vi "SelectMessages.vi"(8 "error in (no error)":errorcluster, 11 "Messages in":T1[](array[typedef])) -> (0 "error out":errorcluster, 2 "Cancelled":bool, 3 "Messages out":T1[](array[typedef]))   [LabVIEW 2017, in "MessageGen.lvlib"]
uses:
  <vilib>/addons/InsightCM/MessageBus/CodeGen/MessageGen.lvlib
  <vilib>/addons/InsightCM/MessageBus/CodeGen/controls/MessageData.ctl
  <vilib>/addons/InsightCM/MessageBus/CodeGen/controls/MessageType.ctl
  <vilib>/addons/InsightCM/MessageBus/CodeGen/controls/Parameter.ctl
  <vilib>/addons/InsightCM/MessageBus/CodeGen/controls/ParameterType.ctl
panel:
  in  "DelectAll":bool
  in  "SelectAll":bool
  in  "Cancel":bool
  in  "Ok":bool
  in  "Messages":cluster{"Boolean":bool, "String":string}[](array[cluster])
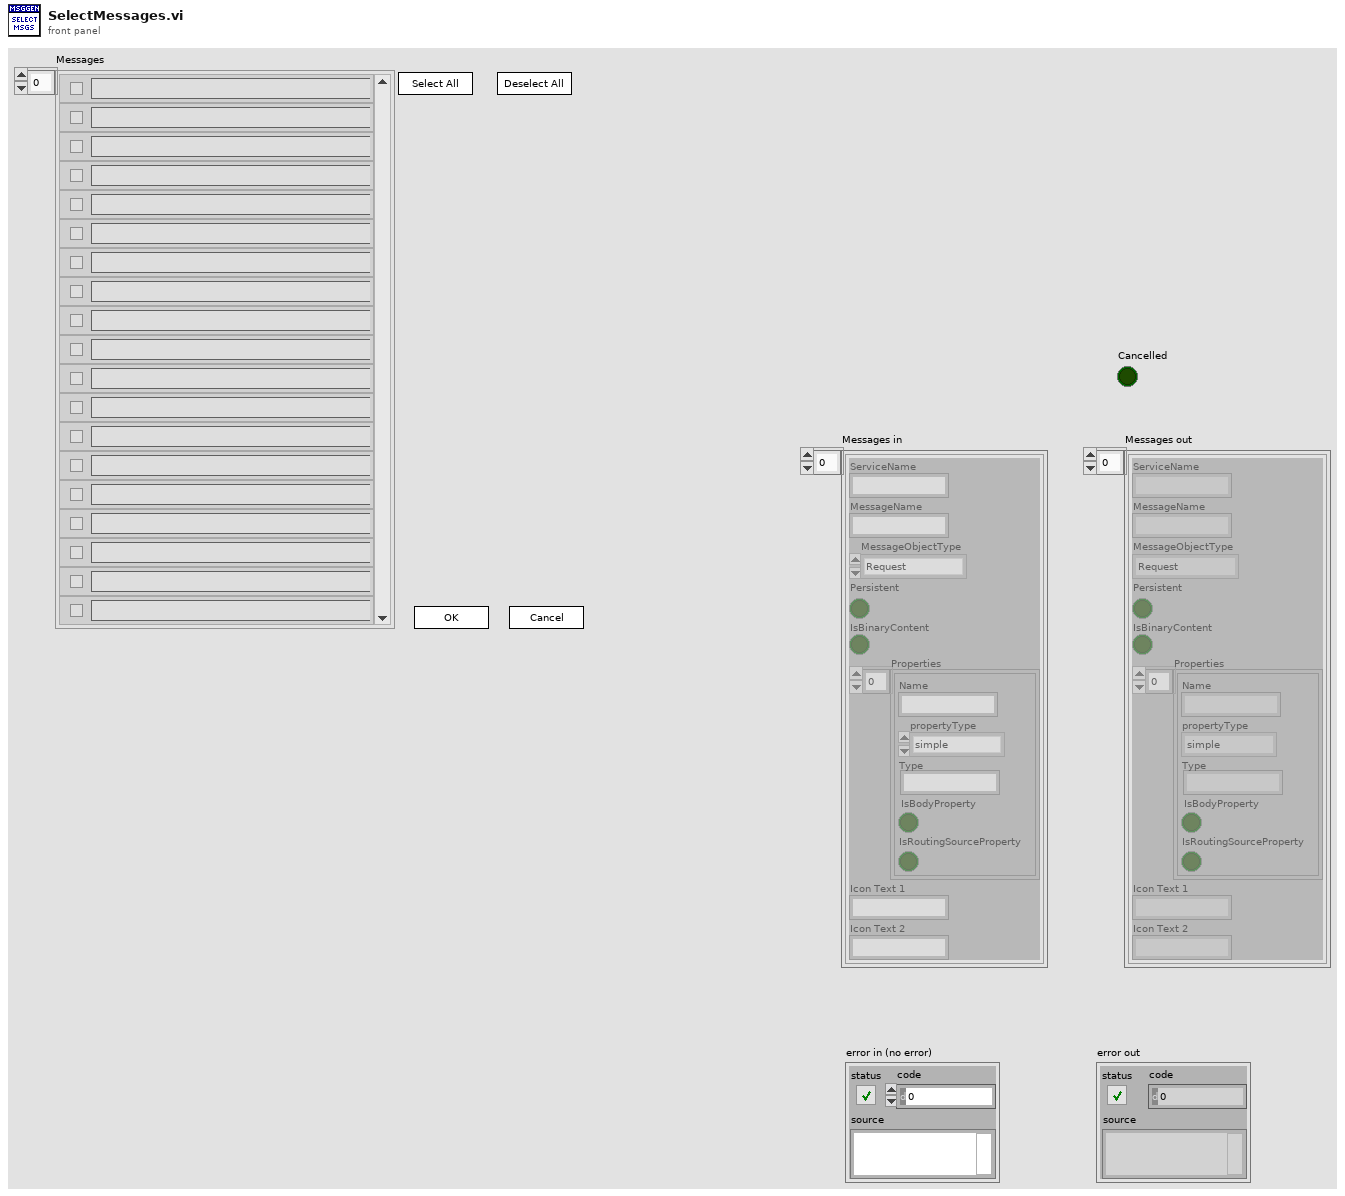
[diagram p1: front panel]
types:
  T1 = typedef "MessageGen.lvlib/MessageData.ctl" = cluster{"ServiceName":string, "MessageName":string, "MessageObjectType":T2, "Persistent":bool, "IsBinaryContent":bool, "Properties":T3[], "Icon Text 1":string, "Icon Text 2":string}
  T2 = typedef "MessageGen.lvlib/MessageType.ctl" = enum16{"Request", "Response", "Broadcast", "RoutedMessage"}
  T3 = typedef "MessageGen.lvlib/Parameter.ctl" = cluster{"Name":string, "propertyType":T4, "Type":string, "IsBodyProperty":bool, "IsRoutingSourceProperty":bool}
  T4 = typedef "MessageGen.lvlib/ParameterType.ctl" = enum16{"simple", "bytearray", "dateTime", "list", "map", "object"}
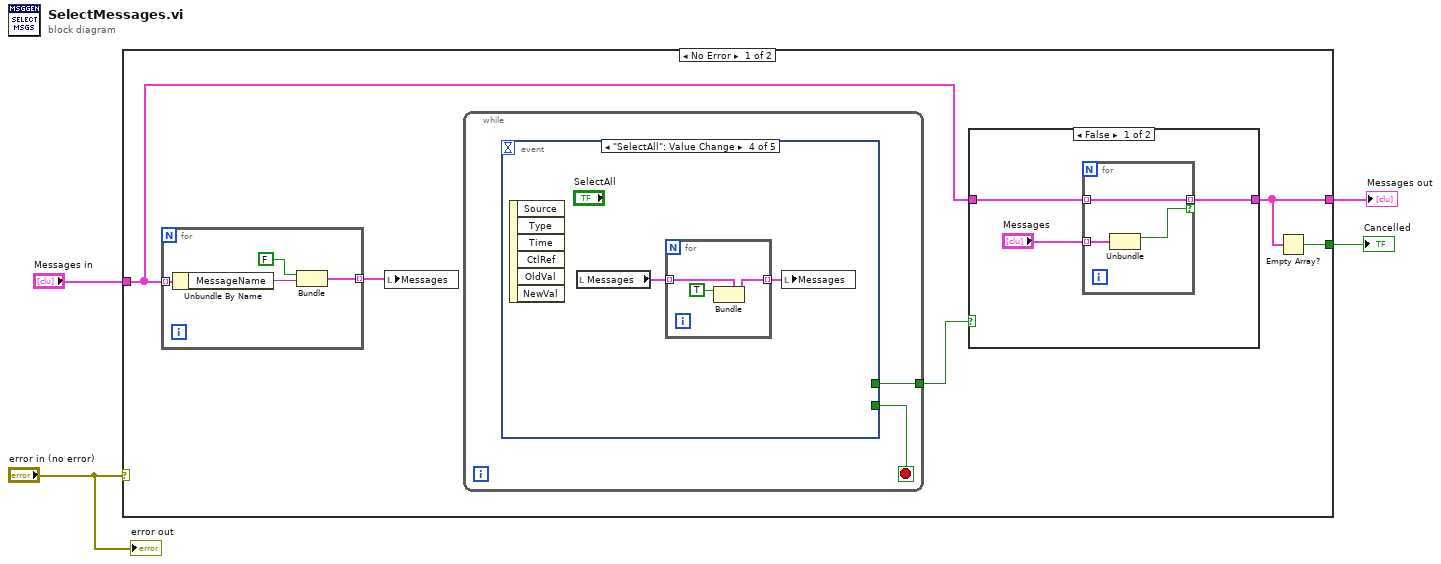
[diagram p0: block diagram]
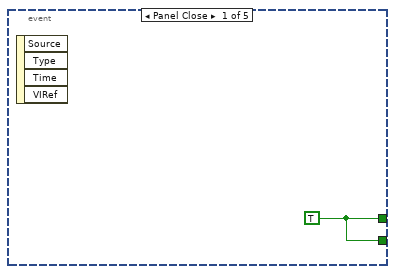
[diagram p3: hidden frame]
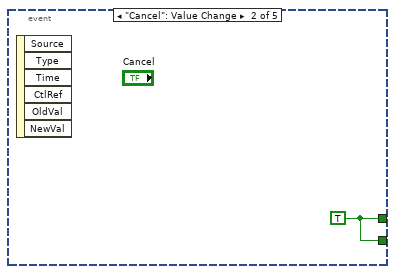
[diagram p4: hidden frame]
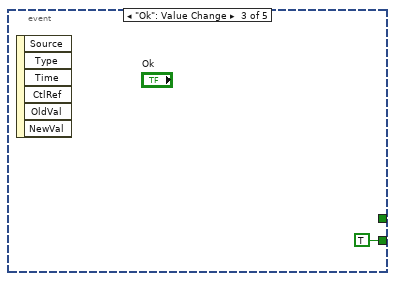
[diagram p5: hidden frame]
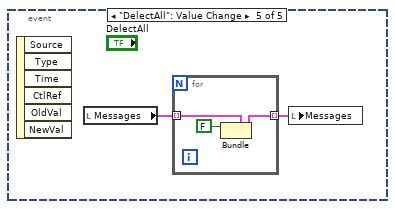
[diagram p6: hidden frame]
diagram:
  n1 = case shown="No Error" "error in (no error)" {
    tunnel: "Messages in" -> [w7 _]
    tunnel: [w6 _] -> w3
    tunnel: [w5 _] -> w2
    frame No Error {
      n2 = for {
        tunnel: w7 -> [w34] mode=indexing
        tunnel: [w31] -> w9 mode=indexing
        n3 = Unbundle By Name(w34) -> ("MessageName"=w33:string)
        n4 = Bundle(FALSE, "MessageName"=w33) -> (w31:cluster{bool, "MessageName":string})  [unwired: 1 in]
      }
      n5 = local write "Messages"(w9) -> ()
      n6 = while {
        tunnel: [w17] -> w8
        stop <- w16 stop-if-true
        n7 = event shown="[3] \"SelectAll\": Value Change" {
          selector: _ -> [_ _ _ _ _]
          dyn-events: _ -> [_ _ _ _ _]
          timeout: _ -> [_ _ _ _ _]
          tunnel: [w18 w19 _ _ _] -> w17
          tunnel: [w18 w19 TRUE _ _] -> w16
          event Panel Close {
            w18 = TRUE
            n8 = event-data() -> ()  [unwired: 1 in, 4 out]
          }
          event "Cancel": Value Change {
            w19 = TRUE
            n9 = event-data() -> ()  [unwired: 1 in, 6 out]
          }
          event "Ok": Value Change {
            n10 = event-data() -> ()  [unwired: 1 in, 6 out]
          }
          event "SelectAll": Value Change {
            n11 = event-data() -> ()  [unwired: 1 in, 6 out]
            n12 = local read "Messages"() -> (w22:cluster{"Boolean":bool, "String":string}[])
            n13 = for {
              tunnel: w22 -> [w23] mode=indexing
              tunnel: [w25] -> w21 mode=indexing
              n14 = Bundle(cluster=w23, "Boolean"=TRUE) -> (w25:cluster{"Boolean":bool, "String":string})  [unwired: 1 in]
            }
            n15 = local write "Messages"(w21) -> ()
          }
          event "DelectAll": Value Change {
            n16 = event-data() -> ()  [unwired: 1 in, 6 out]
            n17 = local read "Messages"() -> (w27:cluster{"Boolean":bool, "String":string}[])
            n18 = for {
              tunnel: w27 -> [w28] mode=indexing
              tunnel: [w30] -> w26 mode=indexing
              n19 = Bundle(cluster=w28, "Boolean"=FALSE) -> (w30:cluster{"Boolean":bool, "String":string})  [unwired: 1 in]
            }
            n20 = local write "Messages"(w26) -> ()
          }
        }
      }
      n21 = case shown="False" w8 {
        tunnel: w7 -> [w12 _]
        tunnel: [w10 _] -> w6
        frame False {
          n22 = for {
            tunnel: [w15] -> w10 mode=indexing if=w13
            tunnel: w12 -> [w15] mode=indexing
            tunnel: "Messages" -> [w14] mode=indexing
            n23 = Unbundle(w14) -> ("Boolean"=w13:bool)  [unwired: 1 out]
          }
        }
        frame True {
        }
      }
      n24 = Empty Array?(array=w6) -> (empty?=w5:bool)
    }
    frame Error {
    }
  }
  "Cancelled" <- w2
  "Messages out" <- w3
  "error out" <- "error in (no error)"
